vi "Multiplexer.vi"(4 "Filter (F)":bool, 5 "AC (F) (F:Nano, T:Digitizer)":bool, 6 "ShortNano (F)":bool, 7 "Multiplexer (Short DC Nano / Voltmeter)":T1=enum."Short AC Sampler", 8 "error in (no error)":errorcluster) -> (0 "error out":errorcluster)   [LabVIEW 2019, in "ACSVcontrol-driver.lvlib"]
doc: "Set Multiplexer. Filter are integrated in the Multiplexer and will be used for DC application typically. ShortNano will short the Nanovoltmeter and leave all other relays depending on Data for Multiplexer. AC option decides whether you connect a nulldetector or a sampler to PJVS or DUT."
uses:
  ACSVcontrol-driver.lvlib
  Type Definitions/Multiplexer.ctl
  Private/Type definitions/Command.ctl
  Private/Type definitions/Status.ctl
  Private/Globals.vi
  <vilib>/Utility/error.llb/Error Cluster From Error Code.vi
  <vilib>/ErrorRing/Error Ring.xnode
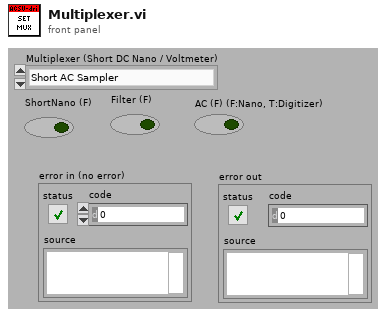
[diagram p1: front panel]
types:
  T1 = typedef "ACSVcontrol-driver.lvlib/Multiplexer.ctl" = enum16{"Short DC Nano / Voltmeter", "Short AC Sampler", "Short Switch DC (JVS->Nano)", "Short Switch AC (JVS->Digit)", "JVS-Voltmeter", "Channel A positive", "Channel A negative", "Channel B positive", "Channel B negative", "Channel C positive", "Channel C negative", "Nulldetector-Channel A+", "Nulldetector-Channel A-", "Nulldetector-Channel B+", "Nulldetector-Channel B-", "Nulldetector-Channel C+", "Nulldetector-Channel C-", "ext.Voltmeter-Channel A+", "ext.Voltmeter-Channel A-", "ext.Voltmeter-Channel B+", "ext.Voltmeter-Channel B-", "ext.Voltmeter-Channel C+", "ext.Voltmeter-Channel C-"}
  T2 = typedef "ACSVcontrol-driver.lvlib/Status.ctl" = enum16{"waiting", "processing", "error command", "Set_PJVS-Done", "Set_Mux-Done", "Set_Mux-Error", "Set_57XX-Done", "Set_57XX-Error", "Set_Gen-Done", "Set_Gen-Error", "Set_Synthesizer-Done", "Set_Synthesizer-Error", "Read_Nano-Done", "Read_Sampler-Done", "Read_Sampler-Error", "Read_Sensors-Done"}
  T3 = typedef "ACSVcontrol-driver.lvlib/Command.ctl" = enum16{"Set_PJVS", "Set_Mux", "Set_57XX", "Set_Gen", "Set_Synthesizer", "Read_Nulldetector", "Read_Sampler", "Read_Sensors"}
  T4 = typedef "ACSVcontrol-driver.lvlib/Timeouts.ctl" = cluster{"TCP Read & Write (ms)":i32, "Sensors readout":i32, "PJVS setup":i32, "Nullmeter readout":i32, "Multiplexer setup":i32, "57XX setup":i32, "Generator setup":i32, "Synthesizer setup":i32, "Sampler readout":i32}
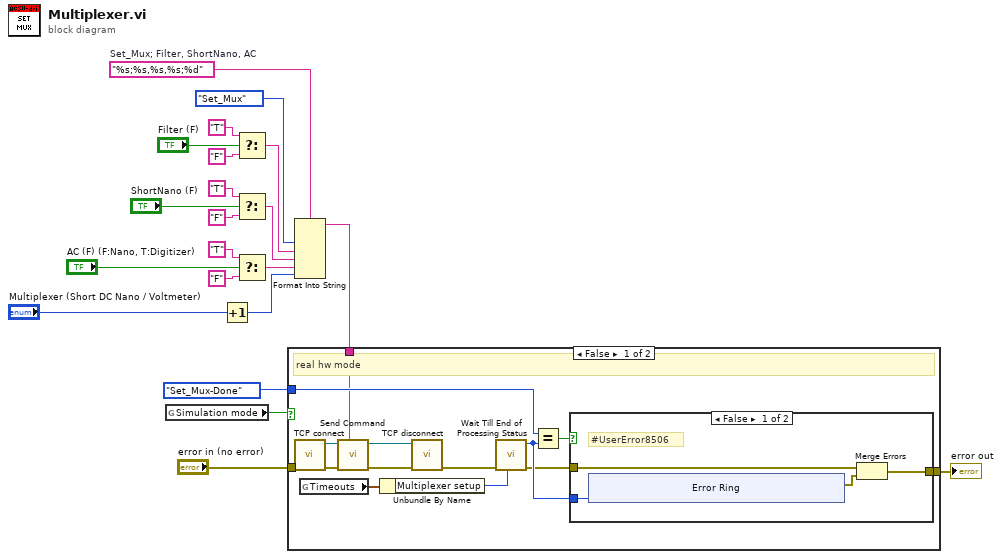
[diagram p0: block diagram]
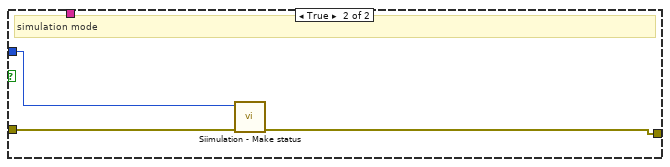
[diagram p3: hidden frame]
diagram:
  w21 = "%s;%s,%s,%s;%d"  # Set_Mux; Filter, ShortNano, AC
  n1 = global read "Globals.vi" "Simulation mode"() -> (w1:bool)
  n2 = Increment(x="Multiplexer (Short DC Nano / Voltmeter)") -> (x+1=w6:T1)
  n3 = Select(t="T" ("format string"), s="Filter (F)", f="F" ("format string")) -> (s? t:f=w10:string)
  n4 = Select(t="T" ("format string"), s="ShortNano (F)", f="F" ("format string")) -> (s? t:f=w9:string)
  n5 = Select(t="T" ("format string"), s="AC (F) (F:Nano, T:Digitizer)", f="F" ("format string")) -> (s? t:f=w8:string)
  n6 = Format Into String(format string=w21, Command."Set_Mux" ("Command"), w10, w9, w8, w6) -> (resulting string=w2:string)  [unwired: 2 in, 1 out]
  n7 = case shown="False" w1 {
    tunnel: "error in (no error)" -> [w35 w50]
    tunnel: Status."Set_Mux-Done" ("x") -> [w27 w48]
    tunnel: [w25 w49] -> w3
    tunnel: w2 -> [w22 _]
    frame False {
      # "real hw mode"
      n8 = call "TCP connect.vi"("error in (no error)"=w35) -> ("error out"=w32:errorcluster, "connection ID"=w31:refnum<k5>)  [unwired: 9 in]
      n9 = global read "Globals.vi" "Timeouts"() -> (w23:T4)
      n10 = call "Send Command.vi"("Command"=w22, "error in (no error)"=w32, "connection ID"=w31) -> ("error out"=w33:errorcluster, "connection ID out"=w34:refnum<k5>)  [unwired: 7 in]
      n11 = Unbundle By Name(w23) -> ("Multiplexer setup"=w24:i32)
      n12 = call "TCP disconnect.vi"("error in (no error)"=w33, "connection ID"=w34) -> ("error out"=w26:errorcluster)  [unwired: 9 in]
      n13 = call "Wait Till End of Processing Status.vi"("Loop Timeout (ms) (5000)"=w24, "error in (no error)"=w26) -> ("error out"=w28:errorcluster, "Last Status"=w30:T2)  [unwired: 8 in]
      n14 = Equal?(x=w27, y=w30) -> (x = y?=w29:bool)
      n15 = case shown="False" w29 {
        tunnel: w28 -> [w39 w47]
        tunnel: [w37 w47] -> w25
        tunnel: w30 -> [w36 _]
        frame False {
          # "#UserError8506"
          n16 = xnode "Error Ring"("parameter 0"=w36) -> ("error out"=w38:errorcluster)
          n17 = Merge Errors(w39, w38) -> (w37:errorcluster)
        }
        frame True {
        }
      }
    }
    frame True {
      # "simulation mode"
      n18 = call "Siimulation - Make status.vi"("error in (no error)"=w50, "Status"=w48) -> ("error out"=w49:errorcluster)  [unwired: 8 in, 1 out]
    }
  }
  "error out" <- w3
